vi "Start.vi"   [LabVIEW 2020, in "OXYGEN_Datastream.lvlib"]
uses:
  OXYGEN_Datastream.lvlib
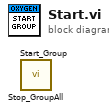
[diagram p0: block diagram]
diagram:
  n1 = call "Stop_GroupAll.vi"() -> ()  [unwired: 9 in, 3 out]
  n2 = call "Start_Group.vi"() -> ()  [unwired: 9 in, 3 out]
